vi "TraverseGetSetups.vi"(2 "Speed Factor":dbl=1.0 min=0.1 max=5.0 format="%.2f", 3 "Traverse Name":string="EnFlo Tunnel") -> (0 "Matched Configurations":T1[](array[typedef]) {"Static Drive Configuration"."Indexer Mode  (FSA)" items=["Incremental", "Absolute"]; "Static Drive Configuration"."Buffer at Stop (SSH)" items=["Clear buffer", "Save and Continue"]; "Static Drive Configuration"."Buffer at Limit (SSG)" items=["Clear buffer", "Save and Continue"]; "Static Drive Configuration"."RS232 Echo Control (SSA)" items=["Echo ON", "Echo OFF"]; "Static Drive Configuration"."Reference edge of Home (OSH)" items=["CW", "CCW"]; "Static Drive Configuration"."Encoder Z for Home (OSD)" items=["Don't use", "Enable"]; "Static Drive Configuration"."Home Switch Sense (OSC)" items=["Normally Open", "Normally Closed"]; "Static Drive Configuration"."Home Position (OSB)" items=["Anywhere in Switch", "Edge of Switch"]; "Static Drive Configuration"."Limit Switch Sense (OSA)" items=["Normally Closed", "Normally Open"]; "Static Drive Configuration"."Limit Disable (LD)" items=["Both Enabled", "CW Disabled", "CCW Disabled", "Both Disabled"]; "Static Drive Configuration"."Stall Detect (FSH)" items=["Disable", "Enable"]; "Static Drive Configuration"."OP2 in Deadband (FSG)" items=["Don't Use", "ACTIVATE"]; "Static Drive Configuration"."Stop on Trigger 3 (FSF)" items=["Ignore", "STOP!"]; "Static Drive Configuration"."Activate OP1 on stall (FSE)" items=["Do not Activate", "ACTIVATE!"]; "Static Drive Configuration"."Stop on Stall (FSD)" items=["Continue", "STOP"]; "Static Drive Configuration"."Position Maintenance (FSC)" items=["Disabled", "Enabled"]; "Static Drive Configuration"."Step Mode  (FSB)" items=["Motor", "Encoder"]; "Static Drive Configuration"."Encoder Resolution (ER)" min=1 max=50000; "Static Drive Configuration"."Dead Band Window (DW)" min=0 max=999999999; "Static Drive Configuration"."Dead Band (DB)" min=0 max=999999999; "Static Drive Configuration"."Correction Gain % (CG)" items=["n/a", "12.5", "25", "37.5", "50", "62.5", "75", "87.5", "100"]; "Channel Properties"."Current Pos" format="%.2f"; "Channel Properties"."Backlash/Eng units" format="%.2f"; "Channel Properties"."Pulses/rev" format="%.2f"; "Channel Properties"."Pos Tolerance" format="%.2f"; "Channel Properties"."Pulses/unit" format="%.2f"; "Channel Properties"."Acc. Min" format="%.2f"; "Channel Properties"."Acc. Max" format="%.2f"; "Channel Properties"."Vel. Min" format="%.2f"; "Channel Properties"."Vel. Max" format="%.2f"; "Channel Properties"."Acc. Default" format="%.2f"; "Channel Properties"."Vel. Default" format="%.2f"})   [LabVIEW 2010]
uses:
  ~subVIs/AxisConfigCluster.ctl
  ~subVIs/DriveProperties.ctl
  ~subVIs/DriveStaticConfig.ctl
  ~subVIs/DriveConfigGlobal.vi
  Anemometry/Anemometry Sub Vis/Globals/Constants_global.vi
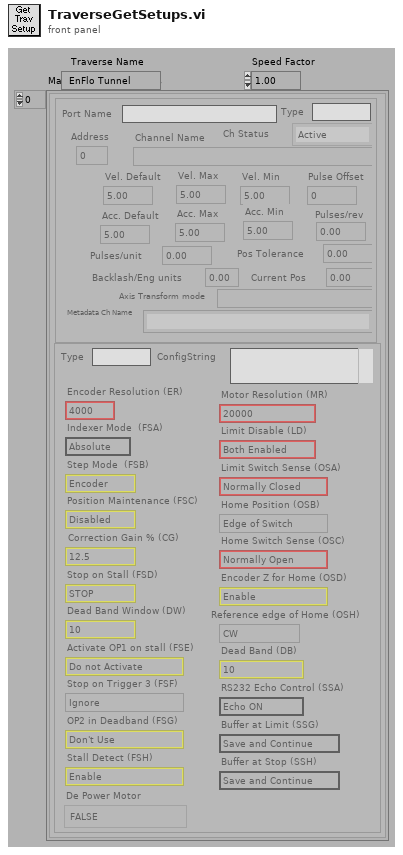
[diagram p1: front panel]
types:
  T1 = typedef "AxisConfigCluster.ctl" = cluster{"Channel Properties":T2, "Static Drive Configuration":T3}
  T2 = typedef "DriveProperties.ctl" = cluster{"Channel Name":string, "Vel. Default":dbl, "Acc. Default":dbl, "Vel. Max":dbl, "Vel. Min":dbl, "Acc. Max":dbl, "Acc. Min":dbl, "Pulses/unit":dbl, "Address":u8, "Pulse Offset":i32, "Pos Tolerance":dbl, "Pulses/rev":dbl, "Backlash/Eng units":dbl, "Current Pos":dbl, "Ch Status":enum16{"Active", "Offline", "Simulate"}, "Port Name":string, "Axis Transform mode":string, "Metadata Ch Name":string, "Type":string}
  T3 = typedef "DriveStaticConfig.ctl" = cluster{"Correction Gain % (CG)":u16, "Dead Band (DB)":i32, "Dead Band Window (DW)":i32, "Encoder Resolution (ER)":i32, "Step Mode  (FSB)":u16, "Position Maintenance (FSC)":u16, "Stop on Stall (FSD)":u16, "Activate OP1 on stall (FSE)":u16, "Stop on Trigger 3 (FSF)":u16, "OP2 in Deadband (FSG)":u16, "Stall Detect (FSH)":u16, "Limit Disable (LD)":u16, "Motor Resolution (MR)":enum16{"200", "400", "1000", "2000", "4000", "5000", "10000", "12800", "18000", "20000", "21600", "25000", "25400", "25600", "36000", "50000", "278528", "425984", "507904", "614400", "655360", "819200", "1024000"}, "Limit Switch Sense (OSA)":u16, "Home Position (OSB)":u16, "Home Switch Sense (OSC)":u16, "Encoder Z for Home (OSD)":u16, "Reference edge of Home (OSH)":u16, "RS232 Echo Control (SSA)":u16, "Buffer at Limit (SSG)":u16, "Buffer at Stop (SSH)":u16, "Indexer Mode  (FSA)":u16, "Type":string, "ConfigString":string, "De Power Motor":enum16{"TRUE", "FALSE"}}
  T4 = enum16{"Load setup from excel file", "Save setup to excel file"}
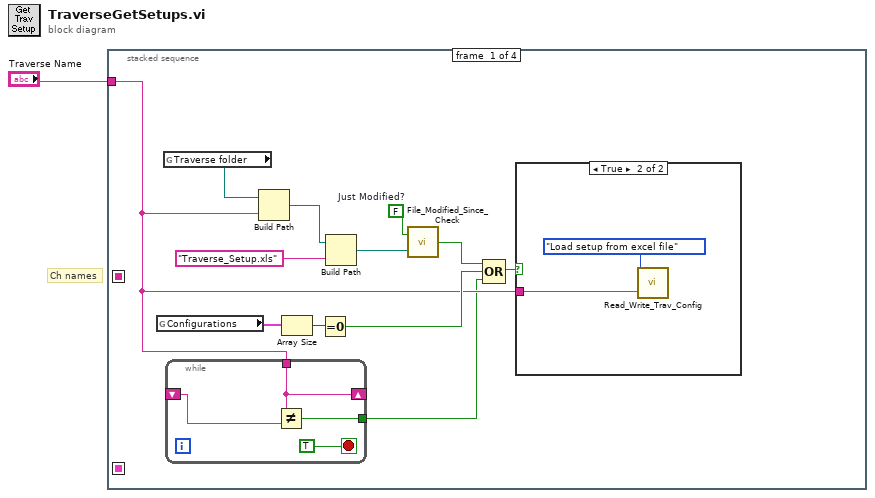
[diagram p0: block diagram]
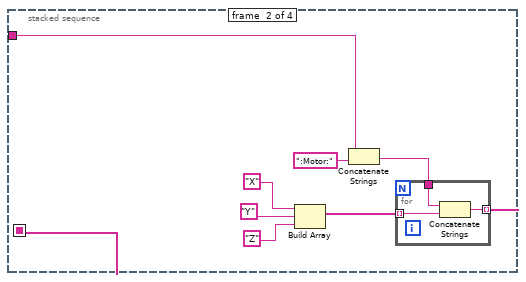
[diagram p3: hidden frame]
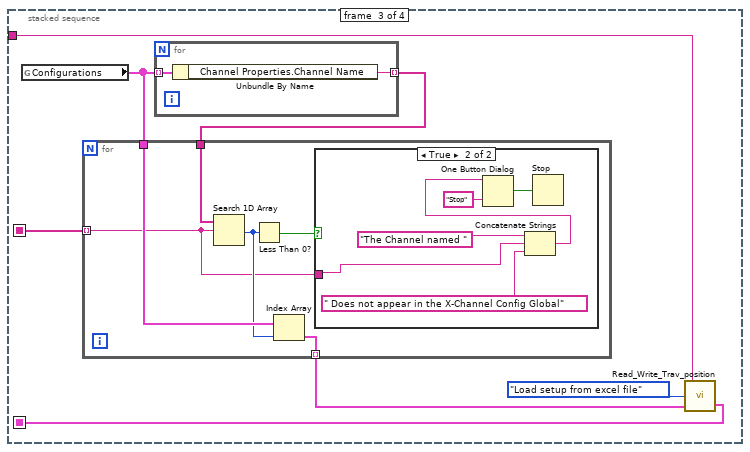
[diagram p4: hidden frame]
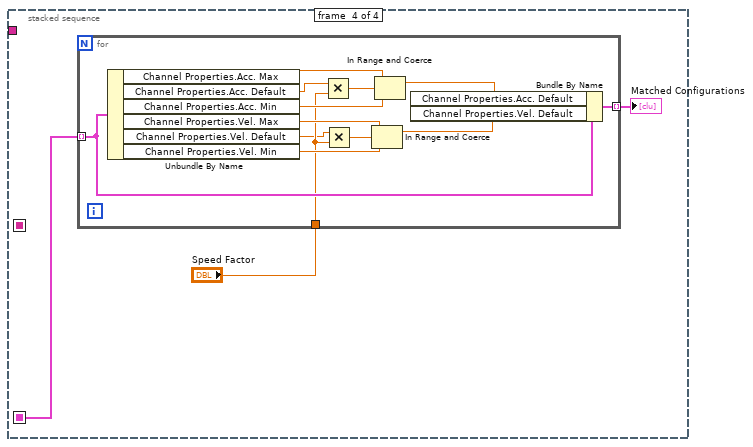
[diagram p6: hidden frame]
diagram:
  # "Ch names"
  n1 = stacked-sequence {
    seq-local: [_ w25 _ _] -> [_ _ w36 _]
    seq-local: [_ _ w33 _] -> [_ _ _ w54]
    tunnel: "Traverse Name" -> [w3 w23 w32 _]
    frame #0 {
      w12 = FALSE  # Just Modified?
      n2 = global read "DriveConfigGlobal.vi" "Configurations"() -> (w11:T1[])
      n3 = global read "Constants_global.vi" "Traverse folder"() -> (w5:path)
      n4 = while {
        shift-right: [w15] -> _
        shift-left: _ -> [w16]
        tunnel: w3 -> [w15]
        tunnel: [w14] -> w2
        stop <- TRUE stop-if-true
        n5 = Not Equal?(x=w15, y=w16) -> (x != y?=w14:bool)
      }
      n6 = Build Path(base path=w5, name or relative path=w3) -> (appended path=w4:path)
      n7 = Array Size(array=w11) -> (size(s)=w10:i32)
      n8 = Equal To 0?(x=w10) -> (x = 0?=w8:bool)
      n9 = Build Path(base path=w4, name or relative path="Traverse_Setup.xls" ("Substring")) -> (appended path=w13:path)
      n10 = call "File_Modified_Since_Check.vi"("Pathname"=w13, "Just Modified?"=w12) -> ("Modified?"=w9:bool)
      n11 = Compound Arithmetic op=OR(w9, w8, w2) -> (w7:bool)
      n12 = case shown="True" w7 {
        tunnel: w3 -> [_ w18]
        frame False {
        }
        frame True {
          n13 = call "Read_Write_Trav_Config.vi"("Traverse Name"=w18, "Mode"=T4."Load setup from excel file") -> ()  [unwired: 1 out]
        }
      }
    }
    frame #1 {
      n14 = Build Array("X", "Y", "Z") -> (w26:string[])
      n15 = Concatenate Strings(w23, ":Motor:") -> (w24:string)
      n16 = for {
        tunnel: w26 -> [w30] mode=indexing
        tunnel: [w28] -> w25 mode=indexing
        tunnel: w24 -> [w29]
        n17 = Concatenate Strings(w29, w30) -> (w28:string)
      }
    }
    frame #2 {
      n18 = global read "DriveConfigGlobal.vi" "Configurations"() -> (w31:T1[])
      n19 = for {
        tunnel: w31 -> [w51] mode=indexing
        tunnel: [w50] -> w37 mode=indexing
        n20 = Unbundle By Name(w51) -> ("Channel Properties.Channel Name"=w50:string)
      }
      n21 = for {
        tunnel: w37 -> [w43]
        tunnel: w31 -> [w41]
        tunnel: [w39] -> w35 mode=indexing
        tunnel: w36 -> [w38] mode=indexing
        n22 = Search 1D Array(1D array=w43, element=w38) -> (index of element=w40:i32)  [unwired: 1 out]
        n23 = Less Than 0?(x=w40) -> (x < 0?=w42:bool)
        n24 = Index Array(array=w41, index=w40) -> (element=w39:T1)
        n25 = case shown="True" w42 {
          tunnel: w38 -> [_ w48]
          frame False {
          }
          frame True {
            n26 = Concatenate Strings("The Channel named " ("message"), w48, " Does not appear in the X-Channel Config Global" ("Input 3")) -> (w44:string)
            n27 = One Button Dialog(message=w44, button name ("OK")="Stop") -> (true=w45:bool)
            n28 = Stop(stop? (T)=w45) -> ()
          }
        }
      }
      n29 = call "Read_Write_Trav_position.vi"("Matched Configurations In"=w35, "Mode"=T4."Load setup from excel file", "Traverse Name"=w32) -> ("Matched Configurations Out"=w33:T1[])  [unwired: 1 out]
    }
    frame #3 {
      n30 = for {
        tunnel: w54 -> [w65] mode=indexing
        tunnel: "Speed Factor" -> [w59]
        tunnel: [w63] -> w52 mode=indexing
        n31 = Unbundle By Name(w65) -> ("Channel Properties.Acc. Max"=w61:dbl, "Channel Properties.Acc. Default"=w56:dbl, "Channel Properties.Acc. Min"=w60:dbl, "Channel Properties.Vel. Max"=w64:dbl, "Channel Properties.Vel. Default"=w55:dbl, "Channel Properties.Vel. Min"=w67:dbl)
        n32 = Multiply(x=w56, y=w59) -> (x*y=w58:dbl)
        n33 = Multiply(x=w55, y=w59) -> (x*y=w66:dbl)
        n34 = In Range and Coerce(upper limit=w64, x=w66, lower limit=w67) -> (coerced(x)=w62:dbl)  [unwired: 1 out]
        n35 = In Range and Coerce(upper limit=w61, x=w58, lower limit=w60) -> (coerced(x)=w57:dbl)  [unwired: 1 out]
        n36 = Bundle By Name(cluster=w65, "Channel Properties.Acc. Default"=w57, "Channel Properties.Vel. Default"=w62) -> (w63:T1)
      }
      "Matched Configurations" <- w52
    }
  }
